vi "test_DefaultDatatype.vi"() -> ()   [LabVIEW 2013]
uses:
  source/TypeDescriptor/OpenDescriptor.lvlib
panel:
  out "error out":errorcluster
  out "Default":variant
  out "Type":u8 format="%.0x"
  out "data string":string
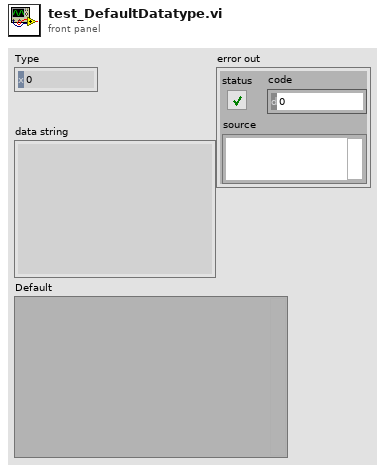
[diagram p1: front panel]
types:
  T1 = cluster{"status":bool, "code":i32, "source":string, "clusterOfIntgers":cluster{i32, i32, i32, i32, i32, i32, i32}, "someEmptyArray":string[]}
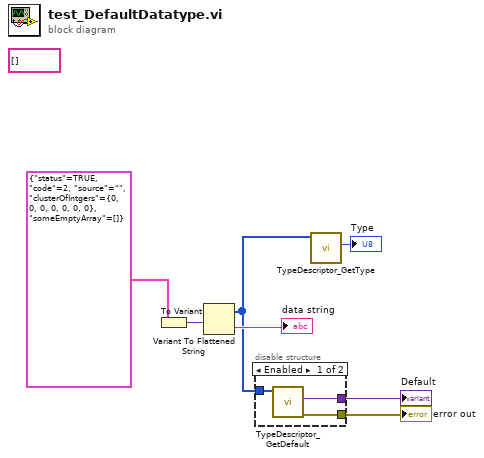
[diagram p0: block diagram]
diagram:
  (unwired) string[] []
  n1 = To Variant(anything=T1 {"status"=TRUE, "code"=2, "source"="", "clusterOfIntgers"={0, 0, 0, 0, 0, 0, 0}, "someEmptyArray"=[]} ("error constant")) -> (Variant=w5:variant)
  n2 = Variant To Flattened String(Variant=w5) -> (data string=→"data string":string, 1:w4:i16[])
  n3 = disable-structure shown="Enabled" {
    disable-tunnel: w4 -> [w10 _]
    disable-tunnel: [w9 _] -> w3
    disable-tunnel: [w8 _] -> w2
    frame Enabled {
      n4 = call "TypeDescriptor_GetDefault.vi"("type descriptor"=w10) -> ("error out"=w8:errorcluster, "Default"=w9:variant)  [unwired: 8 in, 1 out]
    }
    frame Disabled {
    }
  }
  "Default" <- w3
  "error out" <- w2
  n5 = call "TypeDescriptor_GetType.vi"("type descriptor"=w4) -> ("Type"=→"Type":u8)  [unwired: 9 in, 1 out]
